vi "Button Handling.vi"(9 "Array":refnum<vi>[](array[refnum]), 10 "Numeric Array":dbl[](array[numeric]), 11 "Buttons":bool[](array[boolean])) -> ()   [LabVIEW 2017]
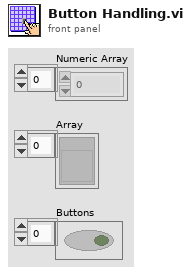
[diagram p1: front panel]
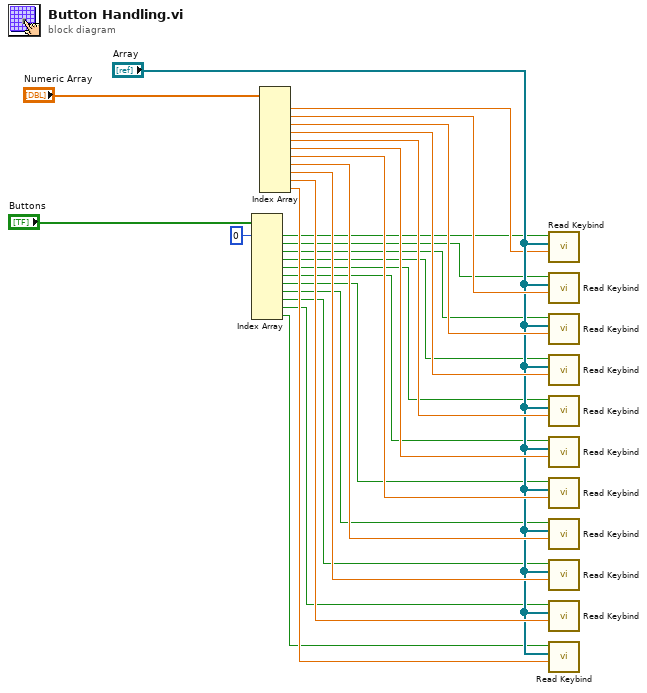
[diagram p0: block diagram]
diagram:
  n1 = Index Array(array="Buttons", index #1=0 ("index")) -> (element #1=w3:bool, element #2=w4:bool, element #3=w5:bool, element #4=w6:bool, element #5=w8:bool, element #6=w9:bool, element #7=w10:bool, element #8=w11:bool, element #9=w12:bool, element #10=w13:bool, element #11=w14:bool)  [unwired: 10 in]
  n2 = Index Array(array="Numeric Array") -> (element #1=w7:dbl, element #2=w16:dbl, element #3=w17:dbl, element #4=w18:dbl, element #5=w19:dbl, element #6=w20:dbl, element #7=w21:dbl, element #8=w22:dbl, element #9=w23:dbl, element #10=w24:dbl, element #11=w25:dbl)  [unwired: 11 in]
  n3 = call "Read Keybind.vi"("Numeric"=w7, "appended array"="Array", "Boolean"=w3) -> ()  [unwired: 9 in]
  n4 = call "Read Keybind.vi"("Numeric"=w16, "appended array"="Array", "Boolean"=w4) -> ()  [unwired: 9 in]
  n5 = call "Read Keybind.vi"("Numeric"=w17, "appended array"="Array", "Boolean"=w5) -> ()  [unwired: 9 in]
  n6 = call "Read Keybind.vi"("Numeric"=w18, "appended array"="Array", "Boolean"=w6) -> ()  [unwired: 9 in]
  n7 = call "Read Keybind.vi"("Numeric"=w19, "appended array"="Array", "Boolean"=w8) -> ()  [unwired: 9 in]
  n8 = call "Read Keybind.vi"("Numeric"=w20, "appended array"="Array", "Boolean"=w9) -> ()  [unwired: 9 in]
  n9 = call "Read Keybind.vi"("Numeric"=w21, "appended array"="Array", "Boolean"=w10) -> ()  [unwired: 9 in]
  n10 = call "Read Keybind.vi"("Numeric"=w22, "appended array"="Array", "Boolean"=w11) -> ()  [unwired: 9 in]
  n11 = call "Read Keybind.vi"("Numeric"=w23, "appended array"="Array", "Boolean"=w12) -> ()  [unwired: 9 in]
  n12 = call "Read Keybind.vi"("Numeric"=w24, "appended array"="Array", "Boolean"=w13) -> ()  [unwired: 9 in]
  n13 = call "Read Keybind.vi"("Numeric"=w25, "appended array"="Array", "Boolean"=w14) -> ()  [unwired: 9 in]
